vi "Drain to ANMB verify dialog.vi"(11 "d":i32=101) -> (3 "Drain?":bool)   [LabVIEW 2019]
panel:
  out "Message 2":string
  out "Message":string
  in  "Cancel Drain":bool
  in  "Start Drain":bool
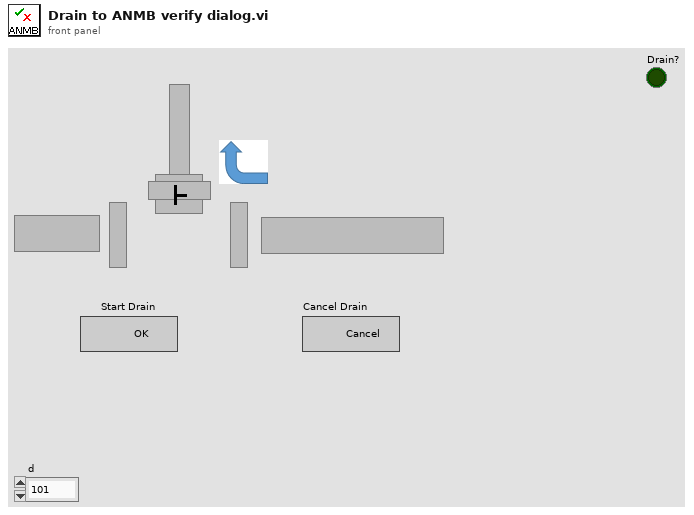
[diagram p1: front panel]
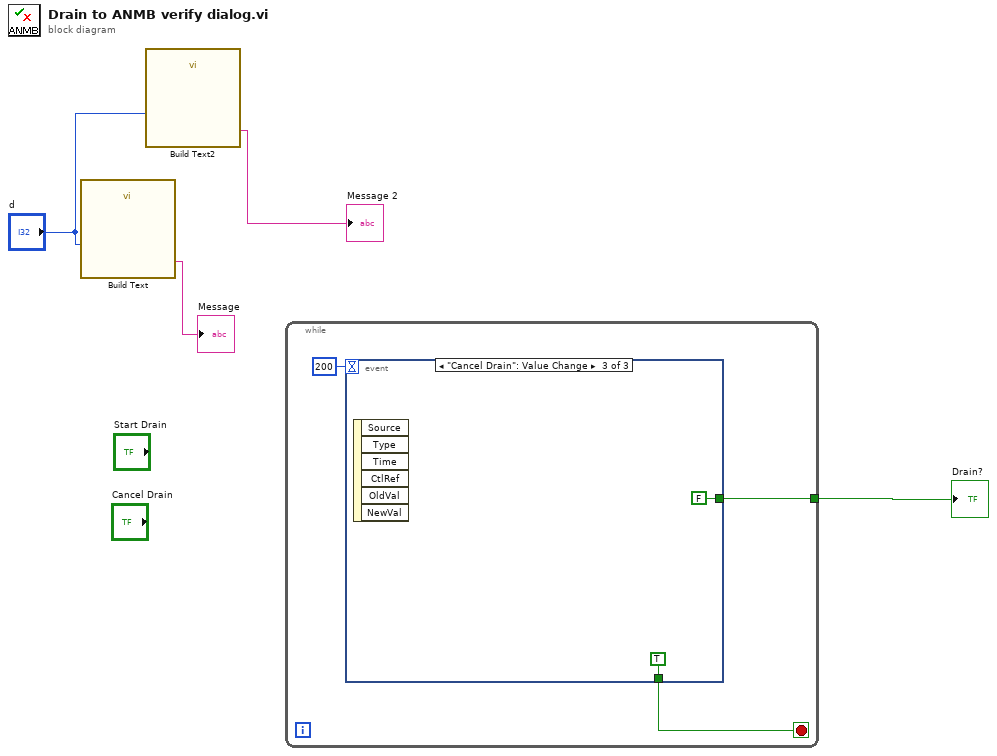
[diagram p0: block diagram]
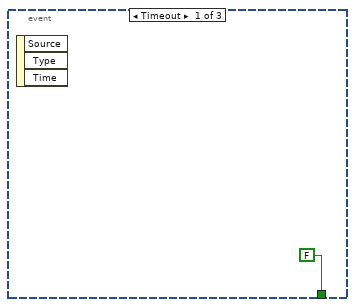
[diagram p2: hidden frame]
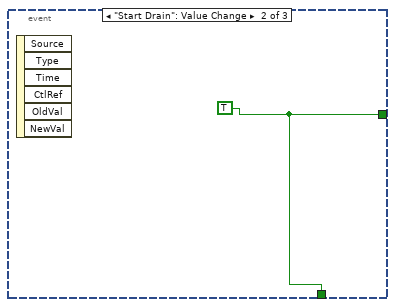
[diagram p3: hidden frame]
diagram:
  n1 = call "Build Text"("d"="d") -> ("Result"=→"Message":string)  [unwired: 13 in, 1 out]
  n2 = call "Build Text2"("d"="d") -> ("Result"=→"Message 2":string)  [unwired: 13 in, 1 out]
  n3 = while {
    tunnel: [w6] -> w4
    stop <- w5 stop-if-true
    n4 = event shown="[2] \"Cancel Drain\": Value Change" {
      selector: _ -> [_ _ _]
      dyn-events: _ -> [_ _ _]
      timeout: 200 -> [_ _ _]
      tunnel: [_ w9 FALSE] -> w6
      tunnel: [FALSE w9 TRUE] -> w5
      event Timeout {
        n5 = event-data() -> ()  [unwired: 1 in, 3 out]
      }
      event "Start Drain": Value Change {
        w9 = TRUE
        n6 = event-data() -> ()  [unwired: 1 in, 6 out]
      }
      event "Cancel Drain": Value Change {
        n7 = event-data() -> ()  [unwired: 1 in, 6 out]
      }
    }
  }
  "Drain?" <- w4
